vi "DHE_set_bpp.vi"(0 "fd":i32, 7 "bpp":i32, 11 "error in (no error)":errorcluster) -> (4 "fd out":i32, 8 "return value":i32, 15 "error out":errorcluster)   [LabVIEW 2016]
doc: "This VI opens (Flag=1) or closes (Flag=0) the instrument shutter."
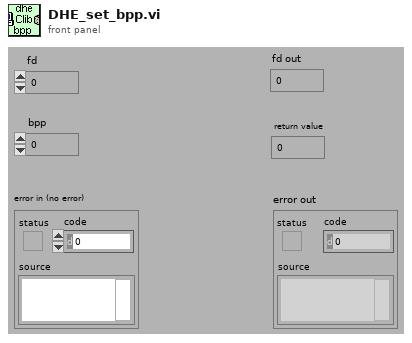
[diagram p1: front panel]
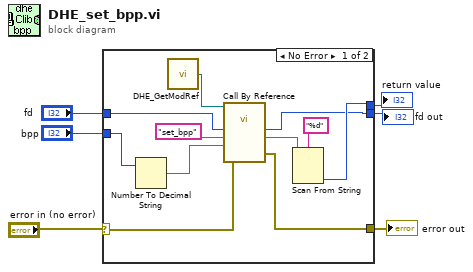
[diagram p0: block diagram]
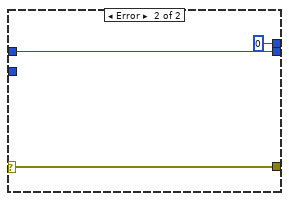
[diagram p2: hidden frame]
diagram:
  n1 = case shown="No Error" "error in (no error)" {
    selector: "error in (no error)" -> [w12 w18]
    tunnel: "fd" -> [w8 w20]
    tunnel: [w10 0] -> w5
    tunnel: [w11 w18] -> w4
    tunnel: "bpp" -> [w7 _]
    tunnel: [w9 w20] -> w2
    frame No Error {
      n2 = Number To Decimal String(number=w7) -> (decimal integer string=w15:string)  [unwired: 1 out]
      n3 = call "DHE_GetModRef.vi"() -> ("DHE_ModRef"=w17:refnum<vi>)  [unwired: 9 out]
      n4 = call-by-ref "?"(reference=w17, "error in (no error)"=w12, "arguments"=w15, "function"="set_bpp", "fd in"=w8) -> ("error out"=w11:errorcluster, "str result"=w14:string, "fd out"=w9:i32)  [unwired: 5 in, 3 out]
      n5 = Scan From String(format string="%d", input string=w14) -> (output 1=w10:i32)  [unwired: 2 in, 4 out]
    }
    frame Error {
    }
  }
  "error out" <- w4
  "return value" <- w5
  "fd out" <- w2
